vi "HIGH_TALK_PH.vi"(0 "Channel":T1, 1 "Port Name":string, 2 "ACTION":enum8{"READ", "INCREASE", "DECREASE", "SET"}(ring), 3 "Main":u8=1 min=1 max=15, 4 "Channel Name":string, 5 "INPUT VALUE":dbl format="%.2f") -> (6 "Comment":string, 7 "OUTPUT VALUE":dbl format="%.2f")   [LabVIEW 2010]
uses:
  ~subvis/Gulton_Channel.ctl
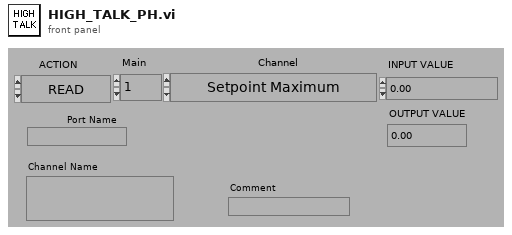
[diagram p1: front panel]
types:
  T1 = typedef "Gulton_Channel.ctl" = enum16{"Setpoint Maximum", "Power Limit", "Limit Comparator Value", "Derivative Term Setting", "Range Maximum", "Range Minimum", "Integral Term Setting", "Status", "MEASURED TEMPERATURE", "Proportional Band Setting", "SETPOINT", "Deviation", "POWER OUTPUT LEVEL"}
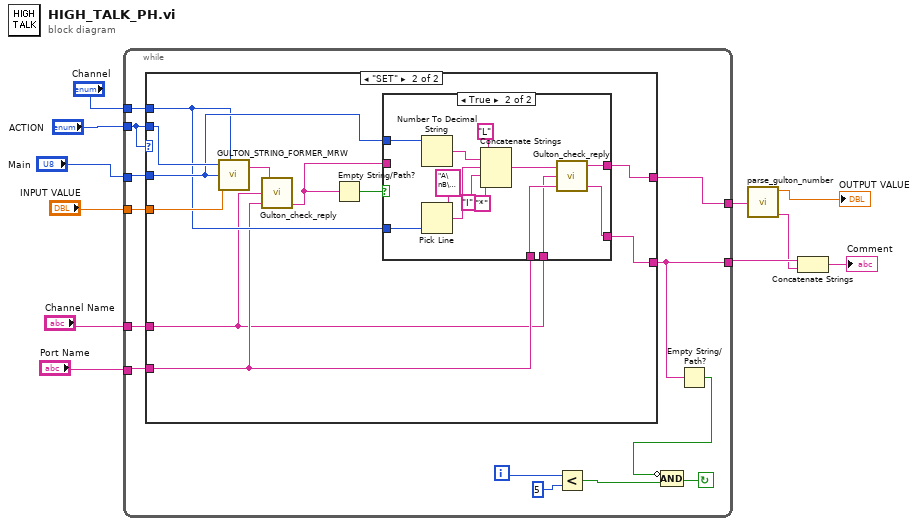
[diagram p0: block diagram]
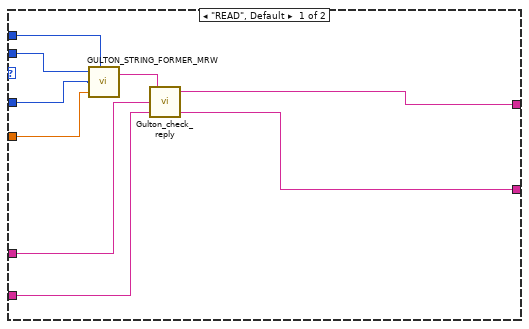
[diagram p2: hidden frame]
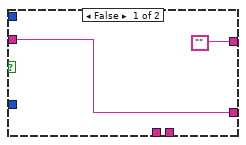
[diagram p3: hidden frame]
diagram:
  n1 = while {
    tunnel: "Channel Name" -> [w13]
    tunnel: [w17] -> w3
    tunnel: [w20] -> w5
    tunnel: "Port Name" -> [w21]
    tunnel: "INPUT VALUE" -> [w22]
    tunnel: "Main" -> [w23]
    tunnel: "ACTION" -> [w12]
    tunnel: "Channel" -> [w24]
    i -> [w18]
    stop <- w14 continue-if-true
    n2 = case shown="\"SET\"" w12 {
      tunnel: w24 -> [w33 w40]
      tunnel: w12 -> [w30 w44]
      tunnel: w23 -> [w29 w41]
      tunnel: w22 -> [w25 w42]
      tunnel: w21 -> [w32 w39]
      tunnel: [w28 w38] -> w20
      tunnel: [w27 w36] -> w17
      tunnel: w13 -> [w26 w34]
      frame "READ", Default {
        n3 = call "GULTON_STRING_FORMER_MRW.vi"("ACTION"=w30, "PARAMETER"=w33, "ZONE"=w29, "INPUT VALUE"=w25) -> ("STRING OUT"=w31:string)  [unwired: 2 in]
        n4 = call "Gulton_check_reply.vi"("Port Name"=w32, "Channel Name"=w26, "Write String"=w31) -> ("Comment out"=w27:string, "Read"=w28:string)  [unwired: 1 in]
      }
      frame "SET" {
        n5 = call "GULTON_STRING_FORMER_MRW.vi"("ACTION"=w44, "PARAMETER"=w40, "ZONE"=w41, "INPUT VALUE"=w42) -> ("STRING OUT"=w43:string)  [unwired: 2 in]
        n6 = call "Gulton_check_reply.vi"("Port Name"=w39, "Channel Name"=w34, "Write String"=w43) -> ("Comment out"=w35:string)  [unwired: 1 in, 1 out]
        n7 = Empty String/Path?(string/path=w35) -> (empty?=w37:bool)
        n8 = case shown="True" w37 {
          tunnel: w41 -> [_ w59]
          tunnel: w40 -> [_ w58]
          tunnel: w39 -> [_ w50]
          tunnel: ["" w49] -> w38
          tunnel: w34 -> [_ w48]
          tunnel: [w45 w47] -> w36
          tunnel: w35 -> [w45 _]
          frame False {
          }
          frame True {
            n9 = Number To Decimal String(number=w59) -> (decimal integer string=w53:string)  [unwired: 1 in]
            n10 = Pick Line(multi-line string="A\nB\nC\nD\nG\nH\nI\nL\nM\nP\nS\nV\nW", line index=w58) -> (output string=w57:string)  [unwired: 1 in]
            n11 = Concatenate Strings("L", w53, w57, "I", "*") -> (w51:string)
            n12 = call "Gulton_check_reply.vi"("Port Name"=w50, "Channel Name"=w48, "Write String"=w51) -> ("Comment out"=w47:string, "Read"=w49:string)  [unwired: 1 in]
          }
        }
      }
    }
    n13 = Less?(x=w18, y=5) -> (x < y?=w16:bool)
    n14 = Empty String/Path?(string/path=w17) -> (empty?=w15:bool)
    n15 = Compound Arithmetic op=AND(invert w15, w16) -> (w14:bool)
  }
  n16 = call "parse_gulton_number.vi"("Stripped Gulton String"=w5) -> ("value"=→"OUTPUT VALUE":dbl, "Error notes"=w2:string)  [unwired: 2 in]
  n17 = Concatenate Strings(w3, w2) -> (→"Comment":string)
